vi "Detector Close.vi"(8 "error in (no error)":errorcluster, 11 "RIMAS Detector in":refnum<class "Obsolete Detector.lvclass">) -> (0 "error out":errorcluster, 3 "RIMAS Detector out":refnum<class "Obsolete Detector.lvclass">)   [LabVIEW 2022 SP3, in "Obsolete Detector.lvclass"]
uses:
  Obsolete Detector.lvclass
  Obsolete Detector.lvclass/Obsolete Detector.ctl
  Detector Class.lvclass
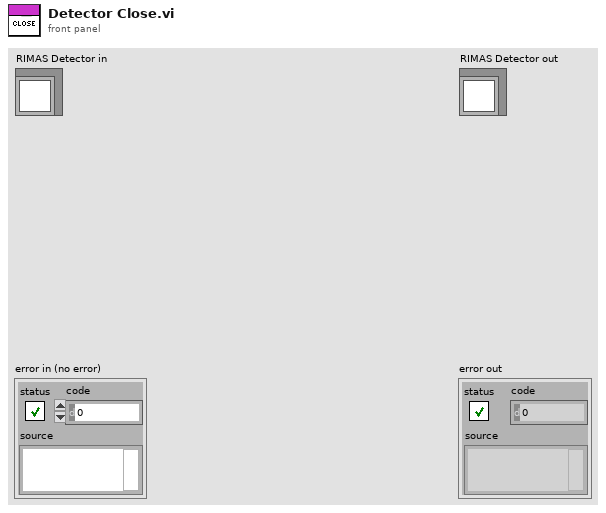
[diagram p1: front panel]
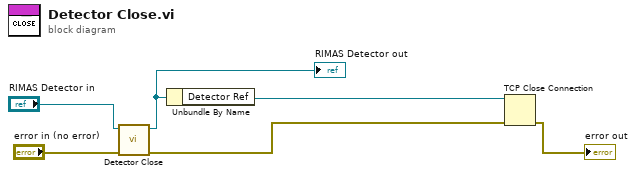
[diagram p0: block diagram]
diagram:
  n1 = call-parent "Detector Close.vi"("error in (no error)"="error in (no error)", "Detector Class in"="RIMAS Detector in") -> ("error out"=w2:errorcluster, "Detector Class out"=w4:refnum<class "Obsolete Detector.lvclass">)  [unwired: 8 in]
  "RIMAS Detector out" <- w4
  n2 = Unbundle By Name(w4) -> ("Detector Ref"=w3:refnum<k5>)
  n3 = TCP Close Connection(connection ID=w3, error in (no error)=w2) -> (error out=→"error out":errorcluster)  [unwired: 1 in, 1 out]
